vi "cg_fid_V1.0.vi"() -> ()   [LabVIEW 2011]
panel:
  out "XY Graph 2":cluster{"Y":dbl[], "Y":dbl[]}[](graph)
  out "Numeric":i32
  in  "start Button":bool
  out "TCD":dbl(graph)
  out "FID":dbl(graph)
  in  "stop":bool
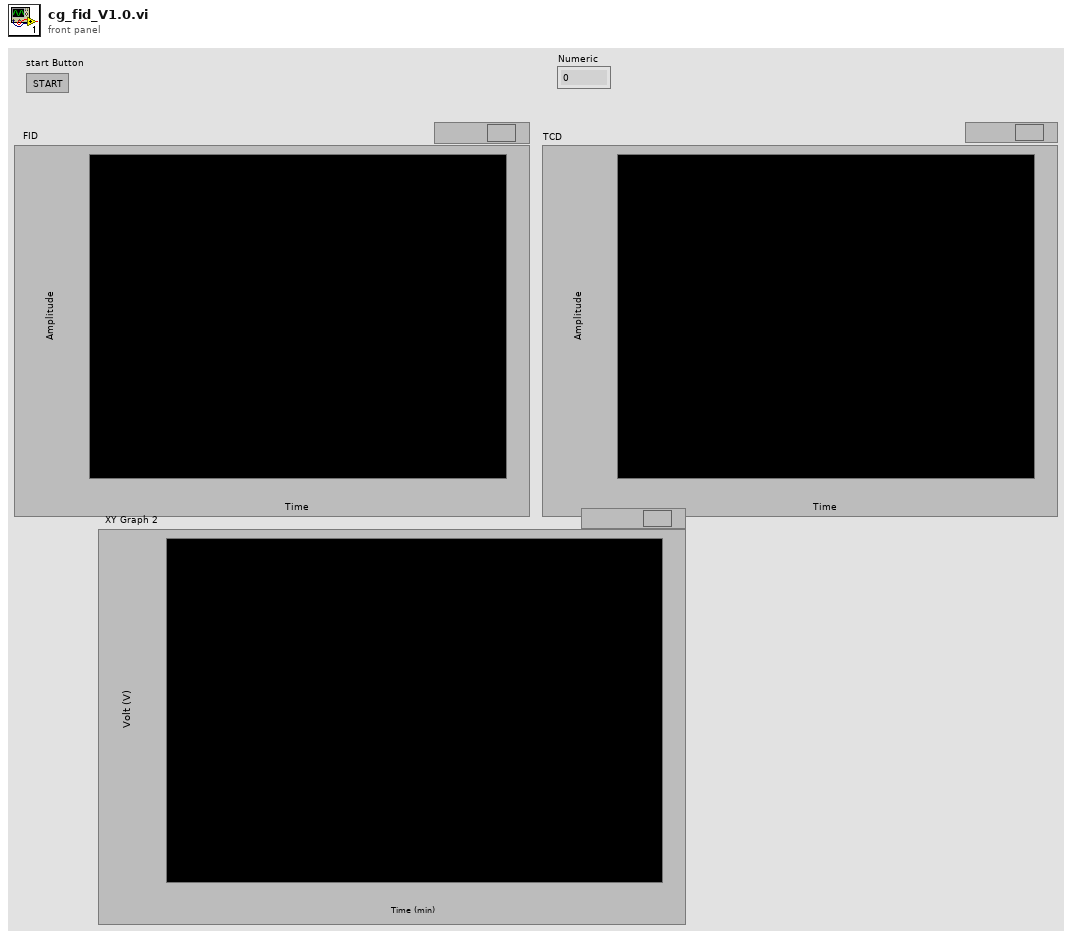
[diagram p1: front panel]
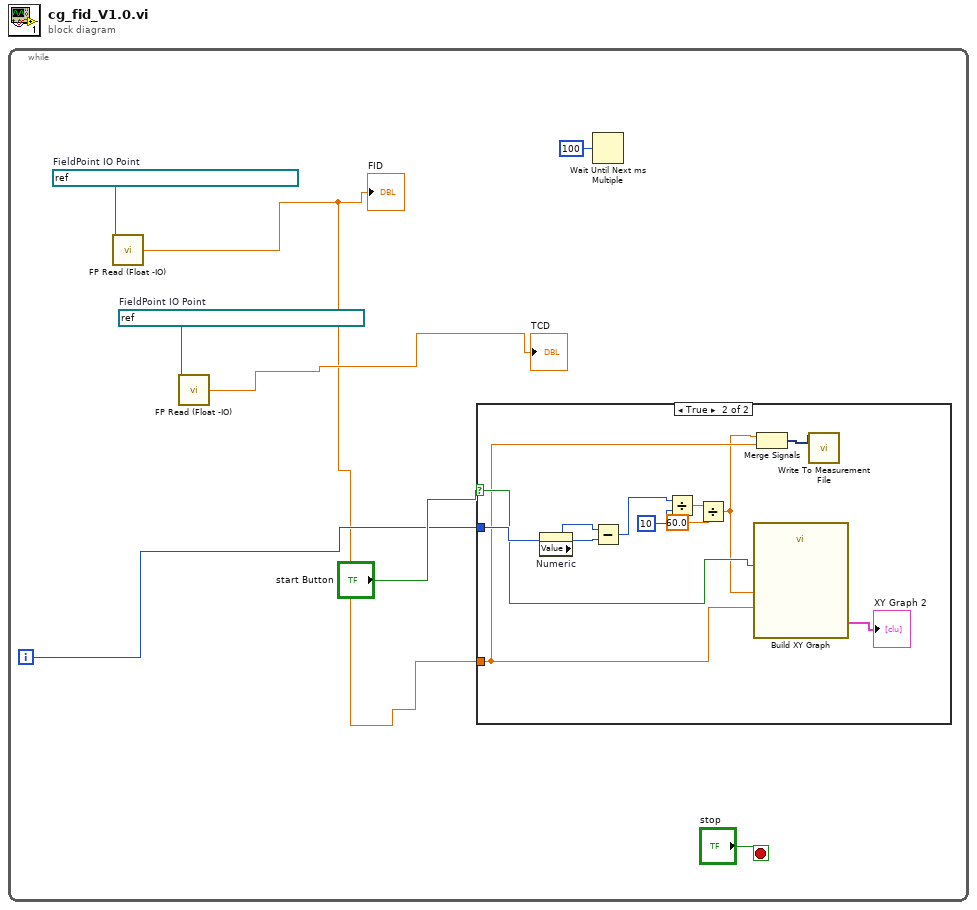
[diagram p0: block diagram]
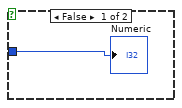
[diagram p2: hidden frame]
diagram:
  n1 = while {
    i -> [w2]
    stop <- "stop" stop-if-true
    w6 = refnum<k21> "FieldPoint\\cfp2220\\cFP-AI-110 @4\\Channel 2"  # FieldPoint IO Point
    w8 = refnum<k21> "FieldPoint\\cfp2220\\cFP-AI-110 @4\\Channel 0"  # FieldPoint IO Point
    n2 = call <vilib>:"FP Read (Float -IO).vi"("FieldPoint IO Point In"=w8) -> ("value"=w1:dbl)  [unwired: 11 in, 3 out]
    "FID" <- w1
    n3 = call <vilib>:"FP Read (Float -IO).vi"("FieldPoint IO Point In"=w6) -> ("value"=→"TCD":dbl)  [unwired: 11 in, 3 out]
    n4 = case shown="True" "start Button" {
      selector: "start Button" -> [_ w12]
      tunnel: w2 -> [w9 w18]
      tunnel: w1 -> [_ w11]
      frame False {
        "Numeric" <- w9
      }
      frame True {
        n5 = property on="Numeric" class="DigNum (strict)"() -> ("Value"=w19:i32)  [unwired: 2 in, 2 out]
        n6 = Subtract(x=w18, y=w19) -> (x-y=w16:i32)
        n7 = Divide(x=w16, y=10) -> (x/y=w14:dbl)
        n8 = Divide(x=w14, y=60.0) -> (x/y=w10:dbl)
        n9 = call "Build XY Graph"("Enable"=w12, "Y Input"=w11, "X Input"=w10) -> ("XY Graph"=→"XY Graph 2":cluster{"Y":dbl[], "Y":dbl[]}[])  [unwired: 2 in, 6 out]
        n10 = Merge Signals(w10, w11) -> (w17:dynamicdata)
        n11 = call "Write To Measurement File"("Signals"=w17) -> ()  [unwired: 16 in, 3 out]
      }
    }
    n12 = Wait Until Next ms Multiple(millisecond multiple=u32 100) -> ()  [unwired: 1 out]
  }
